vi "Open View.vi"(8 "error in (no error)":errorcluster, 9 "Custom Position":cluster{"Top":i16, "Left":i16}, 10 "Position":T1, 11 "IViewable in":refnum<class "IViewable.lvclass">) -> (0 "error out":errorcluster, 3 "IViewable out":refnum<class "IViewable.lvclass">)   [LabVIEW 2015, in "IViewable.lvlib" / "IViewable.lvclass"]
doc: "<License>\nCopyright © 2017 Composed Systems, LLC | All rights reserved\nwww.composed.io\n\nAuthor: Ethan Stern <ethan.stern@composed.io>\n\nThis software is provided \"AS IS\" WITHOUT WARRANTIES, either express or implied, AND IS FOR EDUCATIONAL PURPOSES ONLY.\n</License>"
uses:
  IViewable.lvclass
  View Position Enum.ctl
  IViewable.lvclass/IViewable.ctl
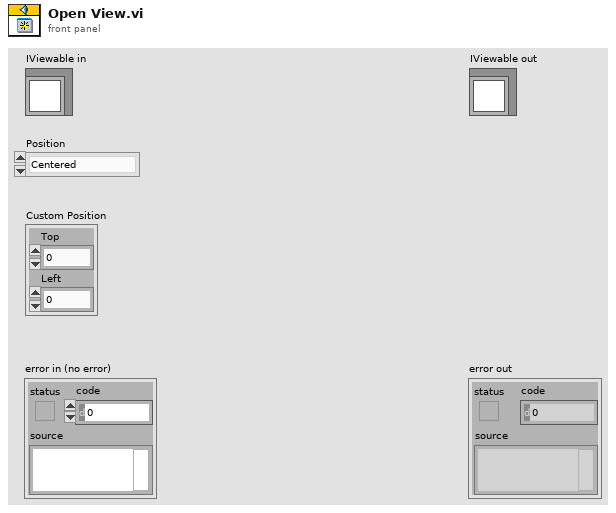
[diagram p1: front panel]
types:
  T1 = typedef "IViewable.lvlib/IViewable.lvclass/View Position Enum.ctl" = enum16{"Centered", "Maximized", "Minimized", "Custom", "Unchanged"}
  T2 = enum32{"Invalid", "Standard", "Closed", "Hidden", "Minimized", "Maximized"}
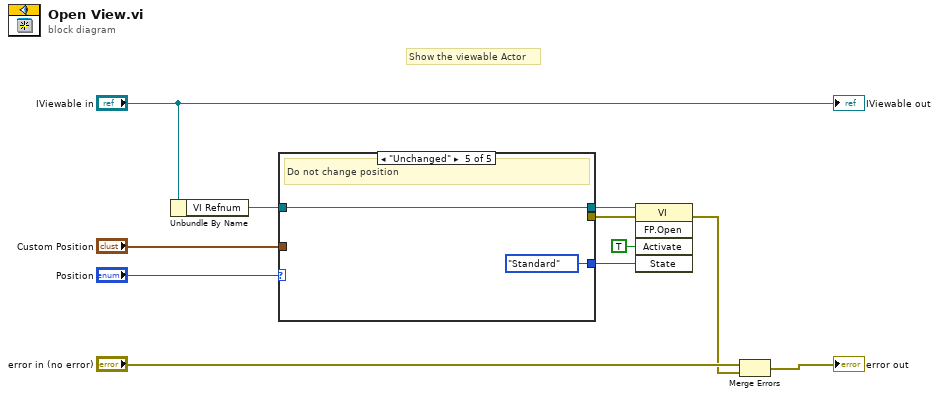
[diagram p0: block diagram]
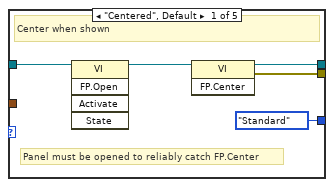
[diagram p2: hidden frame]
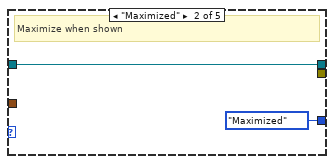
[diagram p3: hidden frame]
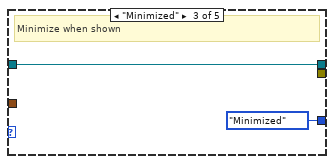
[diagram p4: hidden frame]
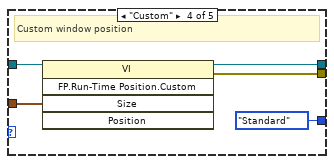
[diagram p5: hidden frame]
diagram:
  # "Show the viewable Actor"
  n1 = Unbundle By Name("IViewable in") -> ("VI Refnum"=w8:refnum<vi>)
  n2 = case shown="\"Unchanged\"" "Position" {
    tunnel: w8 -> [w16 w18 w20 w25 w27]
    tunnel: [w15 w18 w20 w24 w27] -> w4
    tunnel: [w14 _ _ w23 _] -> w3
    tunnel: "Custom Position" -> [_ _ _ w22 _]
    tunnel: [T2."Standard" ("State") T2."Maximized" ("State") T2."Minimized" ("State") T2."Standard" ("State") T2."Standard" ("State")] -> w1
    frame "Centered", Default {
      # "Panel must be opened to reliably catch FP.Center"
      # "Center when shown"
      n3 = invoke class="VI" method="FP.Open"(reference=w16) -> (reference out=w12:refnum<vi>)  [unwired: 4 in, 4 out]
      n4 = invoke class="VI" method="FP.Center"(reference=w12) -> (reference out=w15:refnum<vi>, error out=w14:errorcluster)  [unwired: 2 in, 1 out]
    }
    frame "Maximized" {
      # "Maximize when shown"
    }
    frame "Minimized" {
      # "Minimize when shown"
    }
    frame "Custom" {
      # "Custom window position"
      n5 = invoke class="VI" method="FP.Run-Time Position.Custom"(reference=w25, "Size"=w22) -> (reference out=w24:refnum<vi>, error out=w23:errorcluster)  [unwired: 3 in, 3 out]
    }
    frame "Unchanged" {
      # "Do not change position"
    }
  }
  n6 = invoke class="VI" method="FP.Open"(reference=w4, error in=w3, "Activate"=TRUE ("Activate?"), "State"=w1) -> (error out=w7:errorcluster)  [unwired: 1 in, 4 out]
  n7 = Merge Errors("error in (no error)", w7) -> (→"error out":errorcluster)
  "IViewable out" <- "IViewable in"
